vi "FGV_Speed graph behaviour.vi"(7 "Function":T2, 8 "error in (no error)":errorcluster, 10 "Speed graph behaviour":T1) -> (0 "error out":errorcluster, 2 "Speed graph behaviour":T1)   [LabVIEW 2020]
uses:
  Typedefs/Speed graph behaviour enum.ctl
  Functional Imaging Viewer/Typedefs/Get-Set-Clear Control.ctl
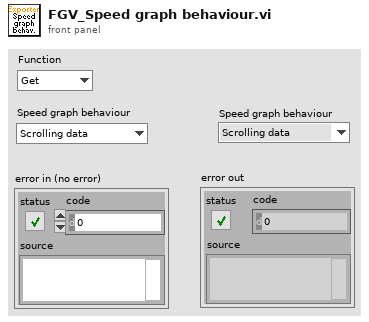
[diagram p1: front panel]
types:
  T1 = typedef "Speed graph behaviour enum.ctl" = enum16{"Scrolling data", "Scrolling cursor"}
  T2 = typedef "Get-Set-Clear Control.ctl" = enum16{"Get", "Set", "Clear"}
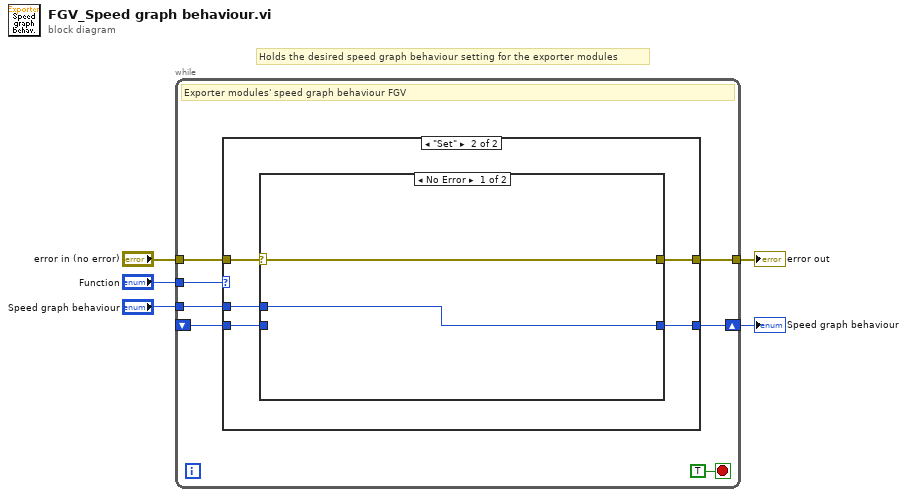
[diagram p0: block diagram]
diagram:
  # "Holds the desired speed graph behaviour setting for the exporter modules"
  n1 = while {
    tunnel: "Speed graph behaviour" -> [w10]
    tunnel: "Function" -> [w11]
    shift-right: [w9] -> w3
    shift-left: _ -> [w8]
    tunnel: "error in (no error)" -> [w7]
    tunnel: [w6] -> w1
    stop <- TRUE stop-if-true
    # "Exporter modules' speed graph behaviour FGV"
    n2 = case shown="\"Set\"" w11 {
      tunnel: w10 -> [_ w16]
      tunnel: [w14 w17] -> w9
      tunnel: w8 -> [w14 w18]
      tunnel: w7 -> [w13 w19]
      tunnel: [w13 w15] -> w6
      frame "Get", Default {
      }
      frame "Set" {
        n3 = case shown="No Error" w19 {
          selector: w19 -> [w20 w22]
          tunnel: w18 -> [_ w23]
          tunnel: [w21 w23] -> w17
          tunnel: w16 -> [w21 _]
          tunnel: [w20 w22] -> w15
          frame No Error {
          }
          frame Error {
          }
        }
      }
    }
  }
  "Speed graph behaviour" <- w3
  "error out" <- w1
